vi "Supplementary Fig.13-2.vi"() -> ()   [LabVIEW 2018]
panel:
  out "files":string[](array[string])
  in  "file type":string=".info"
  in  "filepath":path
  out "diameter [um]":dbl[](array[numeric])
  in  "Cluster":T1={"index"=4, "upper limit"=2.5, "lower limit"=1.0, "Boolean"=TRUE}
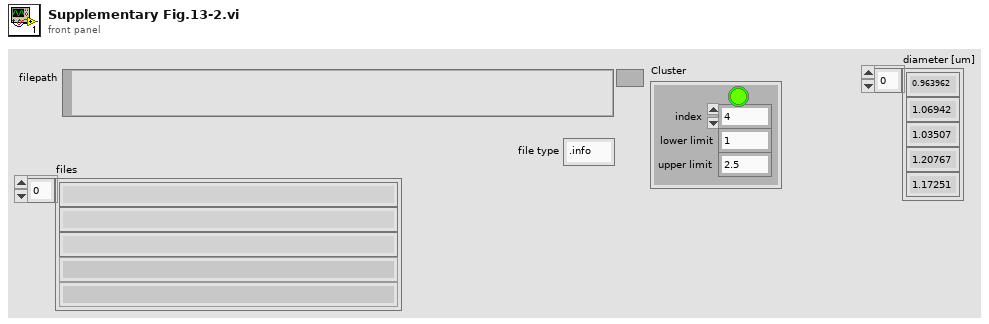
[diagram p1: front panel]
types:
  T1 = cluster{"index":i32, "upper limit":dbl, "lower limit":dbl, "Boolean":bool}
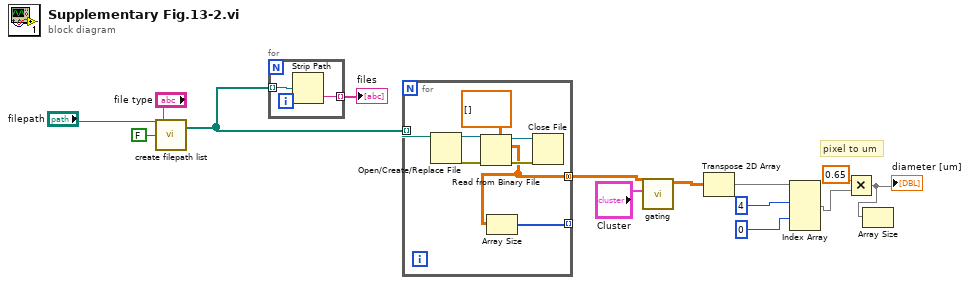
[diagram p0: block diagram]
diagram:
  # "pixel to um"
  n1 = call "create filepath list.vi"("regular expression"="file type", "search subholder"=FALSE, "path"="filepath") -> ("Array"=w2:path[])  [unwired: 1 out]
  n2 = for {
    tunnel: w2 -> [w16] mode=indexing
    tunnel: [w15] -> w3 mode=indexing
    n3 = Strip Path(path=w16) -> (name=w15:string)  [unwired: 1 out]
  }
  "files" <- w3
  n4 = for {
    tunnel: [w18] -> w12 mode=concatenating
    tunnel: w2 -> [w19] mode=indexing
    tunnel: [w17] -> _ mode=indexing
    n5 = Open/Create/Replace File(file path (use dialog)=w19) -> (refnum out=w22:refnum<file>, error out=w21:errorcluster)  [unwired: 5 in, 1 out]
    n6 = Read from Binary File(5:dbl[][] [], 8:w21, 11:w22) -> (0:w24:errorcluster, 2:w18:dbl[][], 3:w23:refnum<file>)  [unwired: 3 in, 1 out]
    n7 = Array Size(array=w18) -> (size(s)=w17:i32[])
    n8 = Close File(refnum=w23, error in=w24) -> ()  [unwired: 2 out]
  }
  n9 = call "gating.vi"("Cluster"="Cluster", "Array in"=w12) -> ("Array out"=w13:dbl[][])  [unwired: 8 in, 1 out]
  n10 = Transpose 2D Array(2D array=w13) -> (transposed array=w7:dbl[][])
  n11 = Index Array(array=w7, index (row) #1=4 ("x"), index (row) #2=0 ("y")) -> (element #1=w11:dbl[])  [unwired: 2 in, 1 out]
  n12 = Multiply(x=0.65, y=w11) -> (x*y=w1:dbl[])
  "diameter [um]" <- w1
  n13 = Array Size(array=w1) -> ()  [unwired: 1 out]
